vi "Energy_GUI.vi"(10 "stop 2":refnum<vi>, 11 "GUI_cluster":T3={"Sub Panel"=refnum, "GUIdevice"="Bella_LP_Mode", "CtlRef"=refnum, "User Event in"=refnum}) -> ()   [LabVIEW 2013]
uses:
  Shared/GUI_Template/GUI_master/tcp new data cluster.ctl
  Controls/eventtypdef1.ctl
  Device Driver/StagingAnalysis/SubVis/energyCalibTypdef.ctl
  <vilib>/Analysis/NI_AALBase.lvlib
  <vilib>/Analysis/1siggen.llb/Ramp Pattern by Samples.vi
  Device Driver/shared/OnOffTypeDef.ctl
  Shared/GUI_Template/GUI_master/tcp_new_data_event.ctl
  Controls/GUI_cluster.ctl
  Device Driver/StagingAnalysis/SubVis/SubVi/polTypDef.ctl
panel:
  in  "Beamselectr":u16(ring) items=["Beam1", "Beam2"]
  in  "tapsselector":u16(ring) items=["Transmission", "Raw Data"]
  in  "Tab Control":enum32{"Transmission", "raw"}(tab)
  out "Chart":dbl(graph) caption="Transmission Beam1"
  out "XY Graph":cluster{"Ramp Pattern":dbl[], "f(X, a)":dbl[]}[](graph)
  in  "plotb calib":bool
  in  "ok::1":T1
  out "Polarization::1":T2
  out "BCaveFilterStatus::1":enum16{"B-Cave filter in", "B-Cave filter out"}(ring)
  in  "EnergyIn::1":dbl caption="Energy in (raw)" min=0.0 max=0.0 format="%#_6p"
  in  "Energy out (raw)::1":dbl caption="Energy out (raw)" min=0.0 max=0.0 format="%#_6p"
  in  "EnergyOut::1":dbl caption="EnergyOut (mJ)" min=0.0 max=0.0 format="%#_6p"
  in  "EnergyTransmission Beam 2::1":dbl caption="Beam 2" min=0.0 max=0.0
  in  "EnergyTransmission Beam 1::1":dbl caption="Beam1" min=0.0 max=0.0
  out "tcp data event":T4
  out "GUIdevice 1":string="Bella_LP_Mode"
  in  "stop":bool
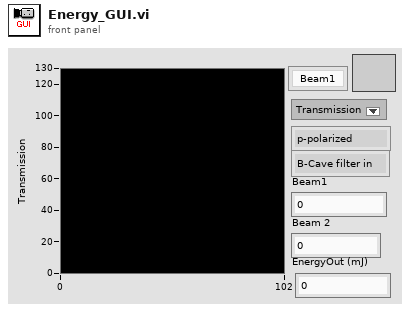
[diagram p1: front panel]
types:
  T1 = typedef "OnOffTypeDef.ctl" = enum16{"off", "on"}
  T2 = typedef "polTypDef.ctl" = enum16{"p-polarized", "s-polarized"}
  T3 = typedef "GUI_cluster.ctl" = cluster{"Sub Panel":refnum<vi>, "GUIdevice":string, "CtlRef":refnum<vi>, "User Event in":refnum<user-event>}
  T4 = typedef "tcp_new_data_event.ctl" = refnum<user-event>
  T5 = typedef "energyCalibTypdef.ctl" = cluster{"p-pol":cluster{"Beam1":dbl, "Beam2":dbl, "Tele":dbl, "startLinear":dbl, "best fit parameters":cluster{"0":dbl, "1":dbl, "2":dbl, "3":dbl}}, "s-pol":cluster{"Beam1":dbl, "Beam2":dbl, "Tele":dbl, "position for fit":dbl, "best fit parameters":cluster{"0":dbl, "1":dbl, "2":dbl, "3":dbl}}, "B-CaveFilter":dbl}
  T6 = typedef "eventtypdef1.ctl" = cluster{"label":string, "Sub Panel":refnum<vi>, "CtlRef":refnum<vi>, "This VI":refnum<vi>}
  T7 = typedef "tcp new data cluster.ctl" = cluster{"EventEnum":enum16{"new data", "connection status update"}, "Device name":string}
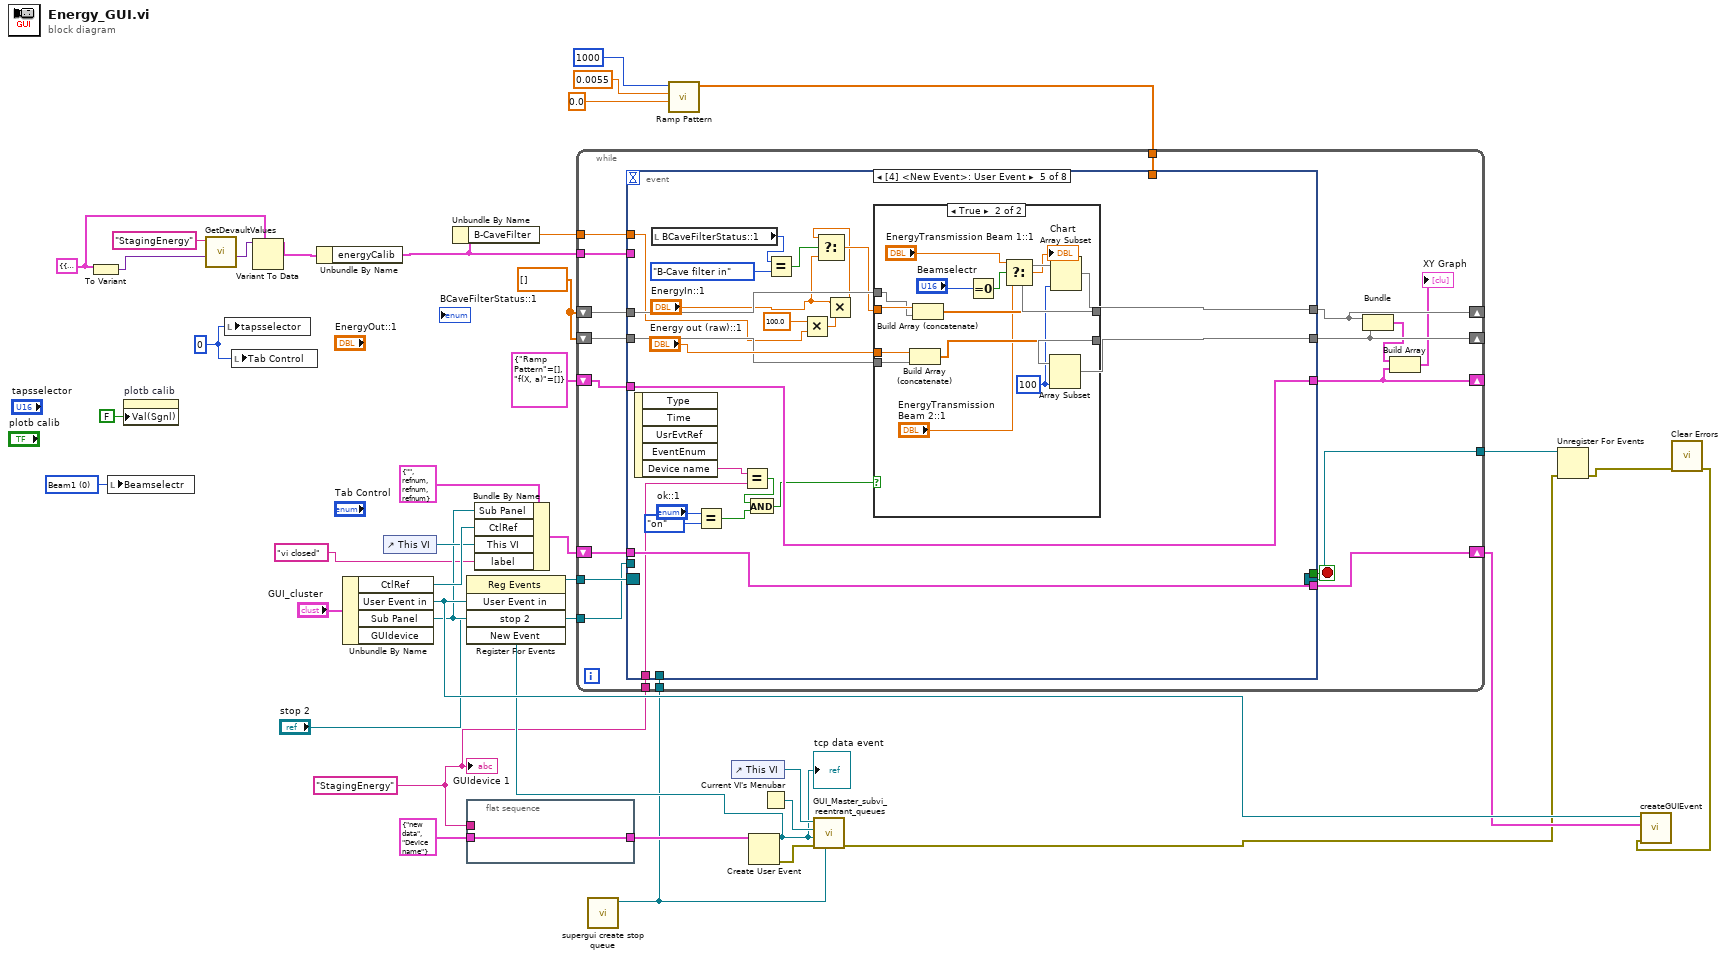
[diagram p0: block diagram]
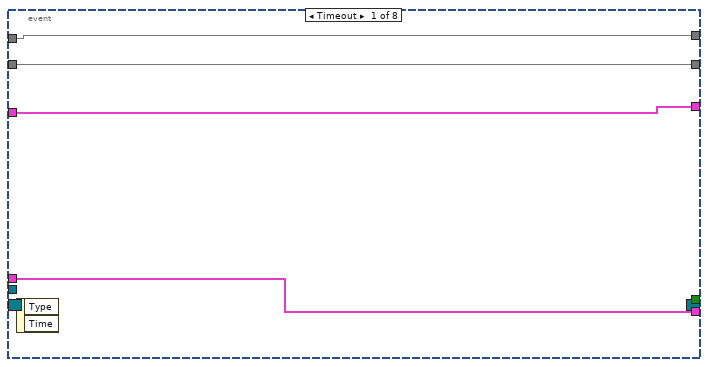
[diagram p2: hidden frame]
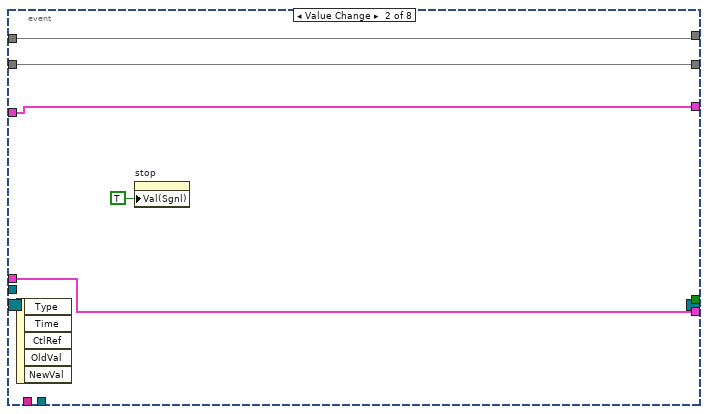
[diagram p3: hidden frame]
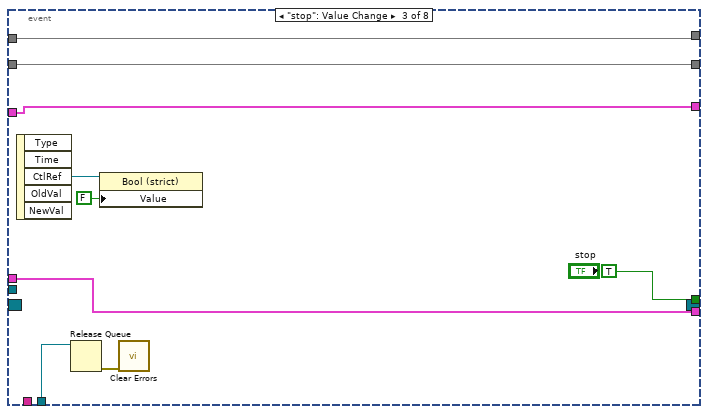
[diagram p4: hidden frame]
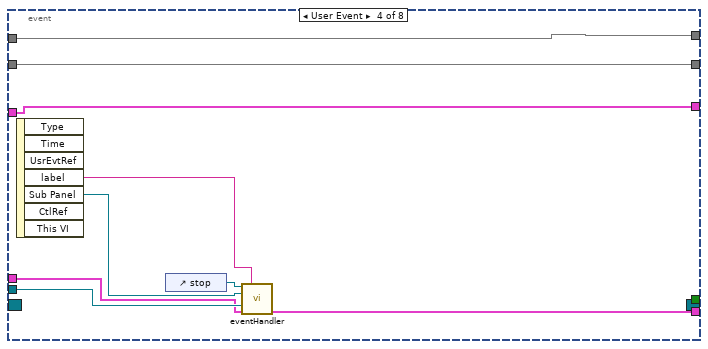
[diagram p5: hidden frame]
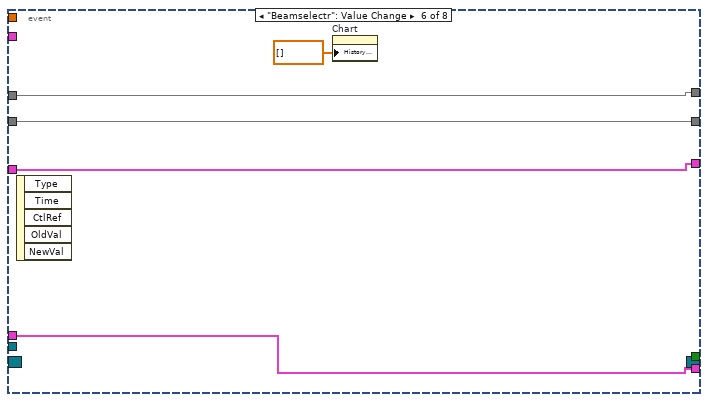
[diagram p7: hidden frame]
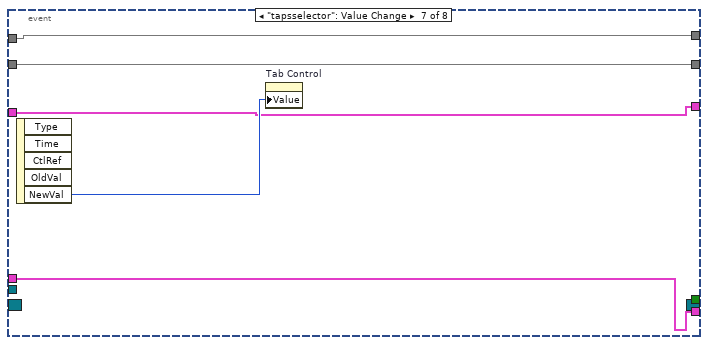
[diagram p8: hidden frame]
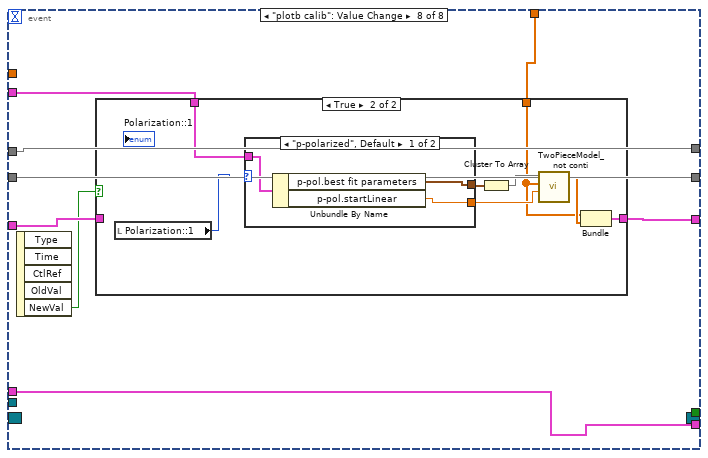
[diagram p9: hidden frame]
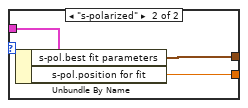
[diagram p11: hidden frame]
diagram:
  w9 = u16 0 items=["Beam1", "Beam2"] ("Beamselectr")
  w10 = 0
  w20 = cluster{"energyCalib":T5} {"energyCalib"={"p-pol"={"Beam1"=0.24495733496510103, "Beam2"=0.755042665034899, "Tele"=0.06901139685565201, "startLinear"=0.0007, "best fit parameters"={"0"=0.06577078607141854, "1"=1075.8816653301244, "2"=-1751262.2505806182, "3"=1069290462.0527091}}, "s-pol"={"Beam1"=0.5855752916708905, "Beam2"=0.4144247083291095, "Tele"=0.004937888283292143, "position for fit"=0.0007, "best fit parameters"={"0"=0.024167, "1"=188.618, "2"=-273128.0, "3"=156332000.0}}, "B-CaveFilter"=0.89}}
  w22 = dbl[] []
  w23 = "StagingEnergy"
  n1 = To Variant(anything=w20) -> (Variant=w17:variant)
  n2 = local write "Beamselectr"(w9) -> ()
  n3 = property on="plotb calib" class="Bool (strict)"("Val(Sgnl)"=FALSE ("Value (Signaling)")) -> ()  [unwired: 2 in, 2 out]
  n4 = call "GetDevaultValues.vi"("variant"=w17, "Device Name"="StagingEnergy") -> ("variant out"=w18:variant)  [unwired: 7 in, 2 out]
  n5 = local write "tapsselector"(w10) -> ()
  n6 = local write "Tab Control"(w10) -> ()
  n7 = Variant To Data(type=w20, Variant=w18) -> (data=w19:cluster{"energyCalib":T5})  [unwired: 1 in, 1 out]
  n8 = Unbundle By Name(w19) -> ("energyCalib"=w7:T5)
  n9 = Unbundle By Name("GUI_cluster") -> ("CtlRef"=w32:refnum<vi>, "User Event in"=w29:refnum<user-event>, "Sub Panel"=w27:refnum<vi>)  [unwired: 1 out]
  n10 = control-ref of="This VI"() -> (w31:refnum<vi>)
  n11 = Unbundle By Name(w7) -> ("B-CaveFilter"=w6:dbl)
  n12 = flat-sequence {
    tunnel: T7 {"EventEnum"=enum."new data", "Device name"="Device name"} ("New Event") -> [w40]
    tunnel: [w40] -> w33
    tunnel: w23 -> [_]
    frame #0 {
    }
  }
  n13 = Bundle By Name(cluster=T6 {"label"="", "Sub Panel"=refnum, "CtlRef"=refnum, "This VI"=refnum} ("event data"), "Sub Panel"=w27, "CtlRef"=w32, "This VI"=w31, "label"="vi closed") -> (w30:T6)
  n14 = call "supergui create stop queue.vi"() -> ("STOP Queue out"=w1:refnum<queue>)  [unwired: 11 in]
  n15 = call-poly <vilib>:"Ramp Pattern.vi"("start"=0.0, "end"=0.0055, "samples"=1000) -> ("Ramp Pattern"=w13:dbl[])  [unwired: 7 in, 1 out]
  n16 = control-ref of="This VI"() -> (w39:refnum<vi>)
  n17 = Create User Event(user event datatype=w33) -> (user event=w24:refnum<user-event>, error out=w37:errorcluster)  [unwired: 1 in]
  "tcp data event" <- w24
  n18 = register-events(w29, "stop 2", w24) -> (reference out=w28:refnum<event-registration>)  [unwired: 2 in, 1 out]
  n19 = while {
    shift-right: [w57] -> w26
    shift-left: w30 -> [w58]
    tunnel: w28 -> [w56]
    tunnel: w27 -> [w55]
    tunnel: w23 -> [w54]
    shift-right: [w51] -> _
    shift-left: w22 -> [w53]
    shift-right: [w50] -> _
    shift-left: w22 -> [w52]
    tunnel: w7 -> [w49]
    tunnel: w13 -> [w48]
    shift-right: [w45] -> _
    shift-left: cluster{"Ramp Pattern":dbl[], "f(X, a)":dbl[]} {"Ramp Pattern"=[], "f(X, a)"=[]} -> [w47]
    tunnel: w6 -> [w43]
    tunnel: [w42] -> w2
    tunnel: w1 -> [w41]
    stop <- w59 stop-if-true
    n20 = event shown="[4] <New Event>: User Event" {
      selector: w56 -> [_ _ _ _ _ _ _ _]
      dyn-events: [_ _ _ _ _ _ _ _] -> w42
      timeout: _ -> [_ _ _ _ _ _ _ _]
      tunnel: [_ _ TRUE ("stop") _ _ _ _ _] -> w59
      tunnel: w58 -> [w63 w68 w77 w83 w112 w127 w132 w141]
      tunnel: [w63 w68 w77 w82 w112 w127 w132 w141] -> w57
      tunnel: w55 -> [_ _ _ w84 _ _ _ _]
      tunnel: w54 -> [_ _ _ _ w110 _ _ _]
      tunnel: [w62 w66 w73 w80 w102 w130 w134 w143] -> w51
      tunnel: w53 -> [w62 w66 w73 w80 w109 w130 w134 w143]
      tunnel: w52 -> [w61 w65 w72 w79 w107 w129 w133 w142]
      tunnel: [w61 w65 w72 w79 w103 w129 w133 w142] -> w50
      tunnel: w49 -> [_ _ _ _ _ _ _ w140]
      tunnel: w48 -> [_ _ _ _ _ _ _ w139]
      tunnel: [w60 w64 w71 w78 w101 w128 w131 w138] -> w45
      tunnel: w47 -> [w60 w64 w71 w78 w101 w128 w131 w137]
      tunnel: w43 -> [_ _ _ _ w91 _ _ _]
      tunnel: w41 -> [_ _ w70 _ _ _ _ _]
      event Timeout {
        n21 = event-data() -> ()  [unwired: 1 in, 2 out]
      }
      event Value Change {
        n22 = event-data() -> ()  [unwired: 1 in, 5 out]
        n23 = property on="stop" class="Bool (strict)"("Val(Sgnl)"=TRUE ("Value (Signaling)")) -> ()  [unwired: 2 in, 2 out]
      }
      event "stop": Value Change {
        n24 = event-data() -> ("CtlRef"=w76:refnum<vi>)  [unwired: 1 in, 4 out]
        n25 = Release Queue(queue=w70) -> (error out=w69:errorcluster)  [unwired: 2 in, 2 out]
        n26 = property class="Bool (strict)"(reference=w76, "Value"=FALSE) -> ()  [unwired: 1 in, 2 out]
        n27 = call <vilib>:"Clear Errors.vi"("error in (no error)"=w69) -> ()  [unwired: 6 in, 1 out]
      }
      event User Event {
        n28 = event-data() -> ("label"=w81:string, "Sub Panel"=w85:refnum<vi>)  [unwired: 1 in, 5 out]
        n29 = control-ref of="stop"() -> (w86:refnum<vi>)
        n30 = call "eventHandler.vi"("Boolean in"=w86, "label"=w81, "Sub Panel 2"=w85, "Sub Panel"=w84, "event data in"=w83) -> ("event data out"=w82:T6)  [unwired: 10 in]
      }
      event User Event {
        w104 = 100 ("length")
        n31 = event-data() -> ("Device name"=w111:string)  [unwired: 1 in, 4 out]
        n32 = local read "BCaveFilterStatus::1"() -> (w95:enum16{"B-Cave filter in", "B-Cave filter out"})
        n33 = Equal?(x="ok::1", y=OnOffTypeDef."on") -> (x = y?=w97:bool)
        n34 = Equal?(x=w111, y=w110) -> (x = y?=w98:bool)
        n35 = And(x=w98, y=w97) -> (x .and. y?=w96:bool)
        n36 = Equal?(x=w95, y=enum16{"B-Cave filter in", "B-Cave filter out"}."B-Cave filter in") -> (x = y?=w93:bool)
        n37 = Multiply(x=100.0, y=w91) -> (x*y=w89:dbl)
        n38 = Multiply(x="EnergyIn::1", y=w89) -> (x*y=w87:dbl)
        n39 = Select(t=w87, s=w93, f="EnergyIn::1") -> (s? t:f=w92:dbl)
        n40 = case shown="True" w96 {
          tunnel: w92 -> [_ w123]
          tunnel: [w114 w125] -> w106
          tunnel: w109 -> [w114 w122]
          tunnel: "Energy out (raw)::1" -> [_ w121]
          tunnel: w107 -> [w113 w120]
          tunnel: [w113 w124] -> w105
          frame False {
          }
          frame True {
            n41 = Build Array (concatenate)(w121, w120) -> (w124:dbl[])
            n42 = Build Array (concatenate)(w123, w122) -> (w125:dbl[])
            n43 = Equal To 0?(x="Beamselectr") -> (x = 0?=w118:bool)
            n44 = Select(t="EnergyTransmission Beam 1::1", s=w118, f="EnergyTransmission Beam 2::1") -> (s? t:f=→"Chart":dbl)
          }
        }
        n45 = Array Subset(array=w105, length=w104) -> (w103:dbl[])  [unwired: 1 in]
        n46 = Array Subset(array=w106, length=w104) -> (w102:dbl[])  [unwired: 1 in]
      }
      event "Beamselectr": Value Change {
        n47 = event-data() -> ()  [unwired: 1 in, 5 out]
        n48 = property on="Chart" class="WFChart (strict)"("History Data"=dbl[] []) -> ()  [unwired: 2 in, 2 out]
      }
      event "tapsselector": Value Change {
        n49 = event-data() -> ("NewVal"=w135:u16)  [unwired: 1 in, 4 out]
        n50 = property on="Tab Control" class="TabCtl (strict)"("Value"=w135) -> ()  [unwired: 2 in, 2 out]
      }
      event "plotb calib": Value Change {
        n51 = event-data() -> ("NewVal"=w136:bool)  [unwired: 1 in, 4 out]
        n52 = case shown="True" w136 {
          tunnel: w140 -> [_ w152]
          tunnel: [w144 w147] -> w138
          tunnel: w139 -> [_ w146]
          tunnel: w137 -> [w144 _]
          frame False {
          }
          frame True {
            n53 = local read "Polarization::1"() -> (w145:T2)
            n54 = case shown="\"p-polarized\", Default" w145 {
              tunnel: w152 -> [w155 w158]
              tunnel: [w154 w157] -> w151
              tunnel: [w153 w156] -> w149
              frame "p-polarized", Default {
                n55 = Unbundle By Name(w155) -> ("p-pol.best fit parameters"=w154:cluster{"0":dbl, "1":dbl, "2":dbl, "3":dbl}, "p-pol.startLinear"=w153:dbl)
              }
              frame "s-polarized" {
                n56 = Unbundle By Name(w158) -> ("s-pol.best fit parameters"=w157:cluster{"0":dbl, "1":dbl, "2":dbl, "3":dbl}, "s-pol.position for fit"=w156:dbl)
              }
            }
            n57 = Cluster To Array(cluster=w151) -> (array=w150:dbl[])
            n58 = call "TwoPieceModel_not conti.vi"("data"=w149, "x"=w146, "a"=w150) -> ("f(X, a)"=w148:dbl[])  [unwired: 1 in, 2 out]
            n59 = Bundle("Ramp Pattern"=w146, "f(X, a)"=w148) -> (w147:cluster{"Ramp Pattern":dbl[], "f(X, a)":dbl[]})  [unwired: 1 in]
          }
        }
      }
    }
    n60 = Bundle(w51, w50) -> (w46:cluster{dbl[], dbl[]})  [unwired: 1 in]
    n61 = Build Array(w46, w45) -> (→"XY Graph":cluster{"Ramp Pattern":dbl[], "f(X, a)":dbl[]}[])
  }
  n62 = Current VI's Menubar() -> (w38:refnum<k9>)
  n63 = call "GUI_Master_subvi_reentrant_queues.vi"("STOP Queue in"=w1, "error in (no error)"=w37, "tcp data event"=w24, "Caller menu reference"=w38, "Caller VI ref"=w39) -> ("error out"=w4:errorcluster)  [unwired: 6 in]
  n64 = Unregister For Events(event registration refnum=w2, error in=w4) -> (error out=w5:errorcluster)
  n65 = call <vilib>:"Clear Errors.vi"("error in (no error)"=w5) -> ("error out"=w3:errorcluster)  [unwired: 6 in]
  n66 = call "createGUIEvent.vi"("error in (no error)"=w3, "event data"=w26, "User Event in"=w29) -> ()  [unwired: 8 in, 1 out]
  "GUIdevice 1" <- w23
